vi "Close.vi"(8 "error in (no error)":errorcluster, 11 "Config-Sqlite in":refnum<class "Config-Sqlite.lvclass">) -> (0 "error out":errorcluster, 3 "Config-Sqlite out":refnum<class "Config-Sqlite.lvclass">)   [LabVIEW 2020, in "CDM-Config.lvlib" / "Config-Sqlite.lvclass"]
uses:
  Config-Sqlite.lvclass
  <vilib>/drjdpowell/SQLite Library/SQL Connection/Connection.lvclass
  Config-Sqlite.lvclass/Config-Sqlite.ctl
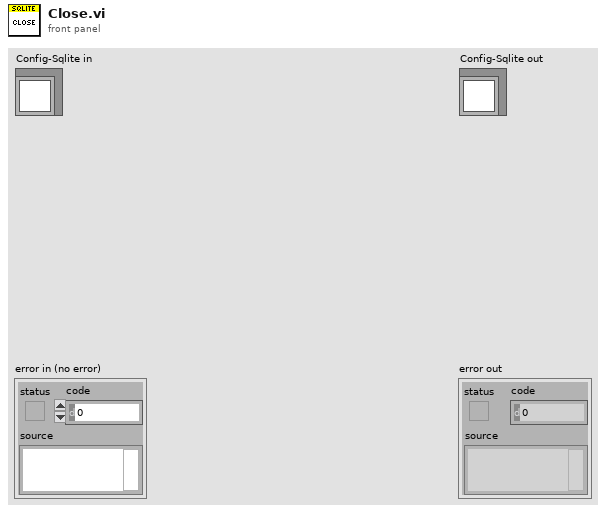
[diagram p1: front panel]
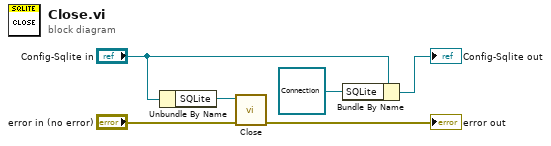
[diagram p0: block diagram]
diagram:
  n1 = Unbundle By Name("Config-Sqlite in") -> ("SQLite"=w5:refnum<class "Connection.lvclass">)
  n2 = call-dynamic "Close.vi"("error in (no error)"="error in (no error)", "SQLite Connection in"=w5) -> ("error out"=→"error out":errorcluster)  [unwired: 9 in]
  n3 = Bundle By Name(cluster="Config-Sqlite in", "SQLite"=refnum<class "Connection.lvclass"> refnum) -> (→"Config-Sqlite out":refnum<class "Config-Sqlite.lvclass">)
